vi "Модификация Витерби.vi"(7 "Кадр с мягкими\nзначениями":dbl[](array[numeric])) -> (8 "Декодированный поток битов":bool[](array[boolean]))   [LabVIEW 2013]
panel:
  in  "Array":cluster{bool, bool}[](array[cluster])=[{TRUE, TRUE}, {TRUE, FALSE}, {FALSE, TRUE}, {FALSE, FALSE}]
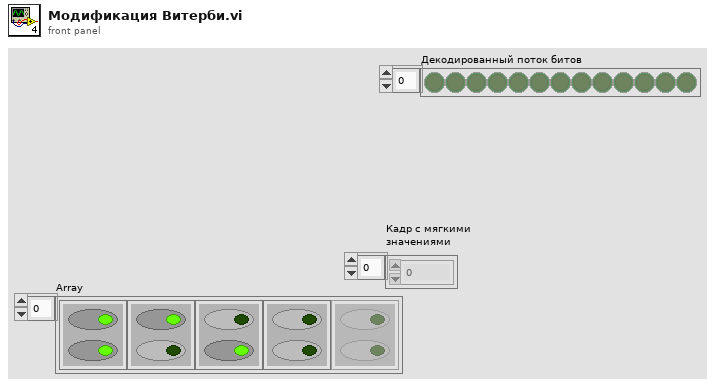
[diagram p1: front panel]
types:
  T1 = cluster{"Пр сост0":i32, "Ном зн\nреб0":i32, "Пр сост1":i32, "Ном зн\nреб1":i32, "Бит":bool}[]
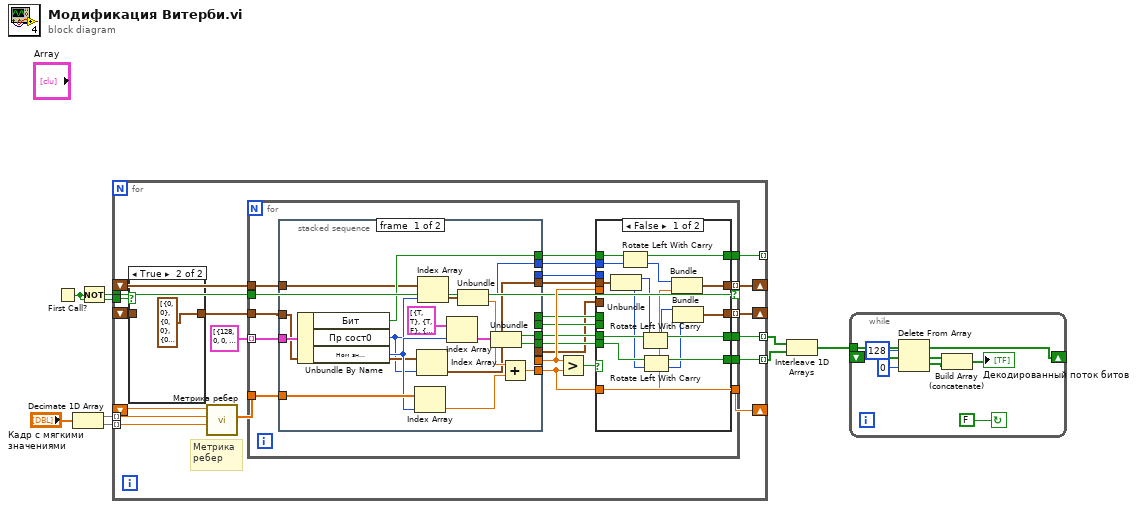
[diagram p0: block diagram]
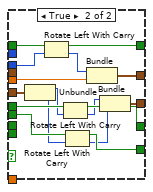
[diagram p3: hidden frame]
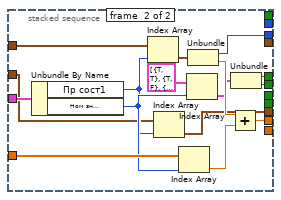
[diagram p4: hidden frame]
diagram:
  n1 = First Call?() -> (First Call?: T/F=w1:bool)
  n2 = Decimate 1D Array("Кадр с мягкими\nзначениями") -> (w7:dbl[], w6:dbl[])
  n3 = Not(x=w1) -> (.not. x?=w5:bool)
  n4 = for {
    tunnel: w7 -> [w18] mode=indexing
    tunnel: w6 -> [w17] mode=indexing
    tunnel: [w23] -> _ mode=indexing
    shift-right: [w22] -> _
    shift-left: _ -> [w21]
    shift-right: [w20] -> _
    shift-left: _ -> [w19]
    tunnel: w5 -> [w15]
    tunnel: [w14] -> w3 mode=indexing
    tunnel: [w13] -> w4 mode=indexing
    shift-right: [w12] -> _
    shift-left: _ -> [w9]
    tunnel: w1 -> [w11]
    # "Метрика\nребер"
    n5 = case shown="True" w11 {
      tunnel: [w25 cluster{u64, u64}[] [{0, 0}, {0, 0}, {0, 0}, {0, 0}, {0, 0}, {0, 0}, {0, 0}, {0, 0}, {0, 0}, {0, 0}, {0, 0}, {0, 0}, {0, 0}, {0, 0}, {0, 0}, {0, 0}, {0, 0}, {0, 0}, {0, 0}, {0, 0}, {0, 0}, {0, 0}, {0, 0}, {0, 0}, {0, 0}, {0, 0}, {0, 0}, {0, 0}, {0, 0}, {0, 0}, {0, 0}, {0, 0}, {0, 0}, {0, 0}, {0, 0}, {0, 0}, {0, 0}, {0, 0}, {0, 0}, {0, 0}, {0, 0}, {0, 0}, {0, 0}, {0, 0}, {0, 0}, {0, 0}, {0, 0}, {0, 0}, {0, 0}, {0, 0}, {0, 0}, {0, 0}, {0, 0}, {0, 0}, {0, 0}, {0, 0}, {0, 0}, {0, 0}, {0, 0}, {0, 0}, {0, 0}, {0, 0}, {0, 0}, {0, 0}, {0, 0}, {0, 0}, {0, 0}, {0, 0}, {0, 0}, {0, 0}, {0, 0}, {0, 0}, {0, 0}, {0, 0}, {0, 0}, {0, 0}, {0, 0}, {0, 0}, {0, 0}, {0, 0}, {0, 0}, {0, 0}, {0, 0}, {0, 0}, {0, 0}, {0, 0}, {0, 0}, {0, 0}, {0, 0}, {0, 0}, {0, 0}, {0, 0}, {0, 0}, {0, 0}, {0, 0}, {0, 0}, {0, 0}, {0, 0}, {0, 0}, {0, 0}, {0, 0}, {0, 0}, {0, 0}, {0, 0}, {0, 0}, {0, 0}, {0, 0}, {0, 0}, {0, 0}, {0, 0}, {0, 0}, {0, 0}, {0, 0}, {0, 0}, {0, 0}, {0, 0}, {0, 0}, {0, 0}, {0, 0}, {0, 0}, {0, 0}, {0, 0}, {0, 0}, {0, 0}, {0, 0}, {0, 0}, {0, 0}, {0, 0}, {0, 0}, {0, 0}, {0, 0}, {0, 0}, {0, 0}, {0, 0}, {0, 0}, {0, 0}, {0, 0}, {0, 0}, {0, 0}, {0, 0}, {0, 0}, {0, 0}, {0, 0}, {0, 0}, {0, 0}, {0, 0}, {0, 0}, {0, 0}, {0, 0}, {0, 0}, {0, 0}, {0, 0}, {0, 0}, {0, 0}, {0, 0}, {0, 0}, {0, 0}, {0, 0}, {0, 0}, {0, 0}, {0, 0}, {0, 0}, {0, 0}, {0, 0}, {0, 0}, {0, 0}, {0, 0}, {0, 0}, {0, 0}, {0, 0}, {0, 0}, {0, 0}, {0, 0}, {0, 0}, {0, 0}, {0, 0}, {0, 0}, {0, 0}, {0, 0}, {0, 0}, {0, 0}, {0, 0}, {0, 0}, {0, 0}, {0, 0}, {0, 0}, {0, 0}, {0, 0}, {0, 0}, {0, 0}, {0, 0}, {0, 0}, {0, 0}, {0, 0}, {0, 0}, {0, 0}, {0, 0}, {0, 0}, {0, 0}, {0, 0}, {0, 0}, {0, 0}, {0, 0}, {0, 0}, {0, 0}, {0, 0}, {0, 0}, {0, 0}, {0, 0}, {0, 0}, {0, 0}, {0, 0}, {0, 0}, {0, 0}, {0, 0}, {0, 0}, {0, 0}, {0, 0}, {0, 0}, {0, 0}, {0, 0}, {0, 0}, {0, 0}, {0, 0}, {0, 0}, {0, 0}, {0, 0}, {0, 0}, {0, 0}, {0, 0}, {0, 0}, {0, 0}, {0, 0}, {0, 0}, {0, 0}, {0, 0}, {0, 0}, {0, 0}, {0, 0}, {0, 0}, {0, 0}, {0, 0}, {0, 0}, {0, 0}, {0, 0}, {0, 0}, {0, 0}, {0, 0}, {0, 0}, {0, 0}, {0, 0}, {0, 0}, {0, 0}, {0, 0}, {0, 0}, {0, 0}]] -> w10
      tunnel: w9 -> [w25 _]
      frame False {
      }
      frame True {
      }
    }
    n6 = call "Метрика ребер.vi"("Бит неч"=w17, "Бит чет"=w18, "ПОРОГ"=w19) -> ("Возможные\nметрики ребер"=w24:dbl[])  [unwired: 8 in]
    n7 = for {
      tunnel: T1 [{"Пр сост0"=128, "Ном зн\nреб0"=0, "Пр сост1"=0, "Ном зн\nреб1"=3, "Бит"=FALSE}, {"Пр сост0"=128, "Ном зн\nреб0"=3, "Пр сост1"=0, "Ном зн\nреб1"=0, "Бит"=TRUE}, {"Пр сост0"=129, "Ном зн\nреб0"=1, "Пр сост1"=1, "Ном зн\nреб1"=2, "Бит"=FALSE}, {"Пр сост0"=129, "Ном зн\nреб0"=2, "Пр сост1"=1, "Ном зн\nреб1"=1, "Бит"=TRUE}, {"Пр сост0"=130, "Ном зн\nреб0"=3, "Пр сост1"=2, "Ном зн\nреб1"=0, "Бит"=FALSE}, {"Пр сост0"=130, "Ном зн\nреб0"=0, "Пр сост1"=2, "Ном зн\nреб1"=3, "Бит"=TRUE}, {"Пр сост0"=131, "Ном зн\nреб0"=2, "Пр сост1"=3, "Ном зн\nреб1"=1, "Бит"=FALSE}, {"Пр сост0"=131, "Ном зн\nреб0"=1, "Пр сост1"=3, "Ном зн\nреб1"=2, "Бит"=TRUE}, {"Пр сост0"=132, "Ном зн\nреб0"=3, "Пр сост1"=4, "Ном зн\nреб1"=0, "Бит"=FALSE}, {"Пр сост0"=132, "Ном зн\nреб0"=0, "Пр сост1"=4, "Ном зн\nреб1"=3, "Бит"=TRUE}, {"Пр сост0"=133, "Ном зн\nреб0"=2, "Пр сост1"=5, "Ном зн\nреб1"=1, "Бит"=FALSE}, {"Пр сост0"=133, "Ном зн\nреб0"=1, "Пр сост1"=5, "Ном зн\nреб1"=2, "Бит"=TRUE}, {"Пр сост0"=134, "Ном зн\nреб0"=0, "Пр сост1"=6, "Ном зн\nреб1"=3, "Бит"=FALSE}, {"Пр сост0"=134, "Ном зн\nреб0"=3, "Пр сост1"=6, "Ном зн\nреб1"=0, "Бит"=TRUE}, {"Пр сост0"=135, "Ном зн\nреб0"=1, "Пр сост1"=7, "Ном зн\nреб1"=2, "Бит"=FALSE}, {"Пр сост0"=135, "Ном зн\nреб0"=2, "Пр сост1"=7, "Ном зн\nреб1"=1, "Бит"=TRUE}, {"Пр сост0"=136, "Ном зн\nреб0"=2, "Пр сост1"=8, "Ном зн\nреб1"=1, "Бит"=FALSE}, {"Пр сост0"=136, "Ном зн\nреб0"=1, "Пр сост1"=8, "Ном зн\nреб1"=2, "Бит"=TRUE}, {"Пр сост0"=137, "Ном зн\nреб0"=3, "Пр сост1"=9, "Ном зн\nреб1"=0, "Бит"=FALSE}, {"Пр сост0"=137, "Ном зн\nреб0"=0, "Пр сост1"=9, "Ном зн\nреб1"=3, "Бит"=TRUE}, {"Пр сост0"=138, "Ном зн\nреб0"=1, "Пр сост1"=10, "Ном зн\nреб1"=2, "Бит"=FALSE}, {"Пр сост0"=138, "Ном зн\nреб0"=2, "Пр сост1"=10, "Ном зн\nреб1"=1, "Бит"=TRUE}, {"Пр сост0"=139, "Ном зн\nреб0"=0, "Пр сост1"=11, "Ном зн\nреб1"=3, "Бит"=FALSE}, {"Пр сост0"=139, "Ном зн\nреб0"=3, "Пр сост1"=11, "Ном зн\nреб1"=0, "Бит"=TRUE}, {"Пр сост0"=140, "Ном зн\nреб0"=1, "Пр сост1"=12, "Ном зн\nреб1"=2, "Бит"=FALSE}, {"Пр сост0"=140, "Ном зн\nреб0"=2, "Пр сост1"=12, "Ном зн\nреб1"=1, "Бит"=TRUE}, {"Пр сост0"=141, "Ном зн\nреб0"=0, "Пр сост1"=13, "Ном зн\nреб1"=3, "Бит"=FALSE}, {"Пр сост0"=141, "Ном зн\nреб0"=3, "Пр сост1"=13, "Ном зн\nреб1"=0, "Бит"=TRUE}, {"Пр сост0"=142, "Ном зн\nреб0"=2, "Пр сост1"=14, "Ном зн\nреб1"=1, "Бит"=FALSE}, {"Пр сост0"=142, "Ном зн\nреб0"=1, "Пр сост1"=14, "Ном зн\nреб1"=2, "Бит"=TRUE}, {"Пр сост0"=143, "Ном зн\nреб0"=3, "Пр сост1"=15, "Ном зн\nреб1"=0, "Бит"=FALSE}, {"Пр сост0"=143, "Ном зн\nреб0"=0, "Пр сост1"=15, "Ном зн\nреб1"=3, "Бит"=TRUE}, {"Пр сост0"=144, "Ном зн\nреб0"=1, "Пр сост1"=16, "Ном зн\nреб1"=2, "Бит"=FALSE}, {"Пр сост0"=144, "Ном зн\nреб0"=2, "Пр сост1"=16, "Ном зн\nреб1"=1, "Бит"=TRUE}, {"Пр сост0"=145, "Ном зн\nреб0"=0, "Пр сост1"=17, "Ном зн\nреб1"=3, "Бит"=FALSE}, {"Пр сост0"=145, "Ном зн\nреб0"=3, "Пр сост1"=17, "Ном зн\nреб1"=0, "Бит"=TRUE}, {"Пр сост0"=146, "Ном зн\nреб0"=2, "Пр сост1"=18, "Ном зн\nреб1"=1, "Бит"=FALSE}, {"Пр сост0"=146, "Ном зн\nреб0"=1, "Пр сост1"=18, "Ном зн\nреб1"=2, "Бит"=TRUE}, {"Пр сост0"=147, "Ном зн\nреб0"=3, "Пр сост1"=19, "Ном зн\nреб1"=0, "Бит"=FALSE}, {"Пр сост0"=147, "Ном зн\nреб0"=0, "Пр сост1"=19, "Ном зн\nреб1"=3, "Бит"=TRUE}, {"Пр сост0"=148, "Ном зн\nреб0"=2, "Пр сост1"=20, "Ном зн\nреб1"=1, "Бит"=FALSE}, {"Пр сост0"=148, "Ном зн\nреб0"=1, "Пр сост1"=20, "Ном зн\nреб1"=2, "Бит"=TRUE}, {"Пр сост0"=149, "Ном зн\nреб0"=3, "Пр сост1"=21, "Ном зн\nреб1"=0, "Бит"=FALSE}, {"Пр сост0"=149, "Ном зн\nреб0"=0, "Пр сост1"=21, "Ном зн\nреб1"=3, "Бит"=TRUE}, {"Пр сост0"=150, "Ном зн\nреб0"=1, "Пр сост1"=22, "Ном зн\nреб1"=2, "Бит"=FALSE}, {"Пр сост0"=150, "Ном зн\nреб0"=2, "Пр сост1"=22, "Ном зн\nреб1"=1, "Бит"=TRUE}, {"Пр сост0"=151, "Ном зн\nреб0"=0, "Пр сост1"=23, "Ном зн\nреб1"=3, "Бит"=FALSE}, {"Пр сост0"=151, "Ном зн\nреб0"=3, "Пр сост1"=23, "Ном зн\nреб1"=0, "Бит"=TRUE}, {"Пр сост0"=152, "Ном зн\nреб0"=3, "Пр сост1"=24, "Ном зн\nреб1"=0, "Бит"=FALSE}, {"Пр сост0"=152, "Ном зн\nреб0"=0, "Пр сост1"=24, "Ном зн\nреб1"=3, "Бит"=TRUE}, {"Пр сост0"=153, "Ном зн\nреб0"=2, "Пр сост1"=25, "Ном зн\nреб1"=1, "Бит"=FALSE}, {"Пр сост0"=153, "Ном зн\nреб0"=1, "Пр сост1"=25, "Ном зн\nреб1"=2, "Бит"=TRUE}, {"Пр сост0"=154, "Ном зн\nреб0"=0, "Пр сост1"=26, "Ном зн\nреб1"=3, "Бит"=FALSE}, {"Пр сост0"=154, "Ном зн\nреб0"=3, "Пр сост1"=26, "Ном зн\nреб1"=0, "Бит"=TRUE}, {"Пр сост0"=155, "Ном зн\nреб0"=1, "Пр сост1"=27, "Ном зн\nреб1"=2, "Бит"=FALSE}, {"Пр сост0"=155, "Ном зн\nреб0"=2, "Пр сост1"=27, "Ном зн\nреб1"=1, "Бит"=TRUE}, {"Пр сост0"=156, "Ном зн\nреб0"=0, "Пр сост1"=28, "Ном зн\nреб1"=3, "Бит"=FALSE}, {"Пр сост0"=156, "Ном зн\nреб0"=3, "Пр сост1"=28, "Ном зн\nреб1"=0, "Бит"=TRUE}, {"Пр сост0"=157, "Ном зн\nреб0"=1, "Пр сост1"=29, "Ном зн\nреб1"=2, "Бит"=FALSE}, {"Пр сост0"=157, "Ном зн\nреб0"=2, "Пр сост1"=29, "Ном зн\nреб1"=1, "Бит"=TRUE}, {"Пр сост0"=158, "Ном зн\nреб0"=3, "Пр сост1"=30, "Ном зн\nреб1"=0, "Бит"=FALSE}, {"Пр сост0"=158, "Ном зн\nреб0"=0, "Пр сост1"=30, "Ном зн\nреб1"=3, "Бит"=TRUE}, {"Пр сост0"=159, "Ном зн\nреб0"=2, "Пр сост1"=31, "Ном зн\nреб1"=1, "Бит"=FALSE}, {"Пр сост0"=159, "Ном зн\nреб0"=1, "Пр сост1"=31, "Ном зн\nреб1"=2, "Бит"=TRUE}, {"Пр сост0"=160, "Ном зн\nреб0"=0, "Пр сост1"=32, "Ном зн\nреб1"=3, "Бит"=FALSE}, {"Пр сост0"=160, "Ном зн\nреб0"=3, "Пр сост1"=32, "Ном зн\nреб1"=0, "Бит"=TRUE}, {"Пр сост0"=161, "Ном зн\nреб0"=1, "Пр сост1"=33, "Ном зн\nреб1"=2, "Бит"=FALSE}, {"Пр сост0"=161, "Ном зн\nреб0"=2, "Пр сост1"=33, "Ном зн\nреб1"=1, "Бит"=TRUE}, {"Пр сост0"=162, "Ном зн\nреб0"=3, "Пр сост1"=34, "Ном зн\nреб1"=0, "Бит"=FALSE}, {"Пр сост0"=162, "Ном зн\nреб0"=0, "Пр сост1"=34, "Ном зн\nреб1"=3, "Бит"=TRUE}, {"Пр сост0"=163, "Ном зн\nреб0"=2, "Пр сост1"=35, "Ном зн\nреб1"=1, "Бит"=FALSE}, {"Пр сост0"=163, "Ном зн\nреб0"=1, "Пр сост1"=35, "Ном зн\nреб1"=2, "Бит"=TRUE}, {"Пр сост0"=164, "Ном зн\nреб0"=3, "Пр сост1"=36, "Ном зн\nреб1"=0, "Бит"=FALSE}, {"Пр сост0"=164, "Ном зн\nреб0"=0, "Пр сост1"=36, "Ном зн\nреб1"=3, "Бит"=TRUE}, {"Пр сост0"=165, "Ном зн\nреб0"=2, "Пр сост1"=37, "Ном зн\nреб1"=1, "Бит"=FALSE}, {"Пр сост0"=165, "Ном зн\nреб0"=1, "Пр сост1"=37, "Ном зн\nреб1"=2, "Бит"=TRUE}, {"Пр сост0"=166, "Ном зн\nреб0"=0, "Пр сост1"=38, "Ном зн\nреб1"=3, "Бит"=FALSE}, {"Пр сост0"=166, "Ном зн\nреб0"=3, "Пр сост1"=38, "Ном зн\nреб1"=0, "Бит"=TRUE}, {"Пр сост0"=167, "Ном зн\nреб0"=1, "Пр сост1"=39, "Ном зн\nреб1"=2, "Бит"=FALSE}, {"Пр сост0"=167, "Ном зн\nреб0"=2, "Пр сост1"=39, "Ном зн\nреб1"=1, "Бит"=TRUE}, {"Пр сост0"=168, "Ном зн\nреб0"=2, "Пр сост1"=40, "Ном зн\nреб1"=1, "Бит"=FALSE}, {"Пр сост0"=168, "Ном зн\nреб0"=1, "Пр сост1"=40, "Ном зн\nреб1"=2, "Бит"=TRUE}, {"Пр сост0"=169, "Ном зн\nреб0"=3, "Пр сост1"=41, "Ном зн\nреб1"=0, "Бит"=FALSE}, {"Пр сост0"=169, "Ном зн\nреб0"=0, "Пр сост1"=41, "Ном зн\nреб1"=3, "Бит"=TRUE}, {"Пр сост0"=170, "Ном зн\nреб0"=1, "Пр сост1"=42, "Ном зн\nреб1"=2, "Бит"=FALSE}, {"Пр сост0"=170, "Ном зн\nреб0"=2, "Пр сост1"=42, "Ном зн\nреб1"=1, "Бит"=TRUE}, {"Пр сост0"=171, "Ном зн\nреб0"=0, "Пр сост1"=43, "Ном зн\nреб1"=3, "Бит"=FALSE}, {"Пр сост0"=171, "Ном зн\nреб0"=3, "Пр сост1"=43, "Ном зн\nреб1"=0, "Бит"=TRUE}, {"Пр сост0"=172, "Ном зн\nреб0"=1, "Пр сост1"=44, "Ном зн\nреб1"=2, "Бит"=FALSE}, {"Пр сост0"=172, "Ном зн\nреб0"=2, "Пр сост1"=44, "Ном зн\nреб1"=1, "Бит"=TRUE}, {"Пр сост0"=173, "Ном зн\nреб0"=0, "Пр сост1"=45, "Ном зн\nреб1"=3, "Бит"=FALSE}, {"Пр сост0"=173, "Ном зн\nреб0"=3, "Пр сост1"=45, "Ном зн\nреб1"=0, "Бит"=TRUE}, {"Пр сост0"=174, "Ном зн\nреб0"=2, "Пр сост1"=46, "Ном зн\nреб1"=1, "Бит"=FALSE}, {"Пр сост0"=174, "Ном зн\nреб0"=1, "Пр сост1"=46, "Ном зн\nреб1"=2, "Бит"=TRUE}, {"Пр сост0"=175, "Ном зн\nреб0"=3, "Пр сост1"=47, "Ном зн\nреб1"=0, "Бит"=FALSE}, {"Пр сост0"=175, "Ном зн\nреб0"=0, "Пр сост1"=47, "Ном зн\nреб1"=3, "Бит"=TRUE}, {"Пр сост0"=176, "Ном зн\nреб0"=1, "Пр сост1"=48, "Ном зн\nреб1"=2, "Бит"=FALSE}, {"Пр сост0"=176, "Ном зн\nреб0"=2, "Пр сост1"=48, "Ном зн\nреб1"=1, "Бит"=TRUE}, {"Пр сост0"=177, "Ном зн\nреб0"=0, "Пр сост1"=49, "Ном зн\nреб1"=3, "Бит"=FALSE}, {"Пр сост0"=177, "Ном зн\nреб0"=3, "Пр сост1"=49, "Ном зн\nреб1"=0, "Бит"=TRUE}, {"Пр сост0"=178, "Ном зн\nреб0"=2, "Пр сост1"=50, "Ном зн\nреб1"=1, "Бит"=FALSE}, {"Пр сост0"=178, "Ном зн\nреб0"=1, "Пр сост1"=50, "Ном зн\nреб1"=2, "Бит"=TRUE}, {"Пр сост0"=179, "Ном зн\nреб0"=3, "Пр сост1"=51, "Ном зн\nреб1"=0, "Бит"=FALSE}, {"Пр сост0"=179, "Ном зн\nреб0"=0, "Пр сост1"=51, "Ном зн\nреб1"=3, "Бит"=TRUE}, {"Пр сост0"=180, "Ном зн\nреб0"=2, "Пр сост1"=52, "Ном зн\nреб1"=1, "Бит"=FALSE}, {"Пр сост0"=180, "Ном зн\nреб0"=1, "Пр сост1"=52, "Ном зн\nреб1"=2, "Бит"=TRUE}, {"Пр сост0"=181, "Ном зн\nреб0"=3, "Пр сост1"=53, "Ном зн\nреб1"=0, "Бит"=FALSE}, {"Пр сост0"=181, "Ном зн\nреб0"=0, "Пр сост1"=53, "Ном зн\nреб1"=3, "Бит"=TRUE}, {"Пр сост0"=182, "Ном зн\nреб0"=1, "Пр сост1"=54, "Ном зн\nреб1"=2, "Бит"=FALSE}, {"Пр сост0"=182, "Ном зн\nреб0"=2, "Пр сост1"=54, "Ном зн\nреб1"=1, "Бит"=TRUE}, {"Пр сост0"=183, "Ном зн\nреб0"=0, "Пр сост1"=55, "Ном зн\nреб1"=3, "Бит"=FALSE}, {"Пр сост0"=183, "Ном зн\nреб0"=3, "Пр сост1"=55, "Ном зн\nреб1"=0, "Бит"=TRUE}, {"Пр сост0"=184, "Ном зн\nреб0"=3, "Пр сост1"=56, "Ном зн\nреб1"=0, "Бит"=FALSE}, {"Пр сост0"=184, "Ном зн\nреб0"=0, "Пр сост1"=56, "Ном зн\nреб1"=3, "Бит"=TRUE}, {"Пр сост0"=185, "Ном зн\nреб0"=2, "Пр сост1"=57, "Ном зн\nреб1"=1, "Бит"=FALSE}, {"Пр сост0"=185, "Ном зн\nреб0"=1, "Пр сост1"=57, "Ном зн\nреб1"=2, "Бит"=TRUE}, {"Пр сост0"=186, "Ном зн\nреб0"=0, "Пр сост1"=58, "Ном зн\nреб1"=3, "Бит"=FALSE}, {"Пр сост0"=186, "Ном зн\nреб0"=3, "Пр сост1"=58, "Ном зн\nреб1"=0, "Бит"=TRUE}, {"Пр сост0"=187, "Ном зн\nреб0"=1, "Пр сост1"=59, "Ном зн\nреб1"=2, "Бит"=FALSE}, {"Пр сост0"=187, "Ном зн\nреб0"=2, "Пр сост1"=59, "Ном зн\nреб1"=1, "Бит"=TRUE}, {"Пр сост0"=188, "Ном зн\nреб0"=0, "Пр сост1"=60, "Ном зн\nреб1"=3, "Бит"=FALSE}, {"Пр сост0"=188, "Ном зн\nреб0"=3, "Пр сост1"=60, "Ном зн\nреб1"=0, "Бит"=TRUE}, {"Пр сост0"=189, "Ном зн\nреб0"=1, "Пр сост1"=61, "Ном зн\nреб1"=2, "Бит"=FALSE}, {"Пр сост0"=189, "Ном зн\nреб0"=2, "Пр сост1"=61, "Ном зн\nреб1"=1, "Бит"=TRUE}, {"Пр сост0"=190, "Ном зн\nреб0"=3, "Пр сост1"=62, "Ном зн\nреб1"=0, "Бит"=FALSE}, {"Пр сост0"=190, "Ном зн\nреб0"=0, "Пр сост1"=62, "Ном зн\nреб1"=3, "Бит"=TRUE}, {"Пр сост0"=191, "Ном зн\nреб0"=2, "Пр сост1"=63, "Ном зн\nреб1"=1, "Бит"=FALSE}, {"Пр сост0"=191, "Ном зн\nреб0"=1, "Пр сост1"=63, "Ном зн\nреб1"=2, "Бит"=TRUE}, {"Пр сост0"=192, "Ном зн\nреб0"=1, "Пр сост1"=64, "Ном зн\nреб1"=2, "Бит"=FALSE}, {"Пр сост0"=192, "Ном зн\nреб0"=2, "Пр сост1"=64, "Ном зн\nреб1"=1, "Бит"=TRUE}, {"Пр сост0"=193, "Ном зн\nреб0"=0, "Пр сост1"=65, "Ном зн\nреб1"=3, "Бит"=FALSE}, {"Пр сост0"=193, "Ном зн\nреб0"=3, "Пр сост1"=65, "Ном зн\nреб1"=0, "Бит"=TRUE}, {"Пр сост0"=194, "Ном зн\nреб0"=2, "Пр сост1"=66, "Ном зн\nреб1"=1, "Бит"=FALSE}, {"Пр сост0"=194, "Ном зн\nреб0"=1, "Пр сост1"=66, "Ном зн\nреб1"=2, "Бит"=TRUE}, {"Пр сост0"=195, "Ном зн\nреб0"=3, "Пр сост1"=67, "Ном зн\nреб1"=0, "Бит"=FALSE}, {"Пр сост0"=195, "Ном зн\nреб0"=0, "Пр сост1"=67, "Ном зн\nреб1"=3, "Бит"=TRUE}, {"Пр сост0"=196, "Ном зн\nреб0"=2, "Пр сост1"=68, "Ном зн\nреб1"=1, "Бит"=FALSE}, {"Пр сост0"=196, "Ном зн\nреб0"=1, "Пр сост1"=68, "Ном зн\nреб1"=2, "Бит"=TRUE}, {"Пр сост0"=197, "Ном зн\nреб0"=3, "Пр сост1"=69, "Ном зн\nреб1"=0, "Бит"=FALSE}, {"Пр сост0"=197, "Ном зн\nреб0"=0, "Пр сост1"=69, "Ном зн\nреб1"=3, "Бит"=TRUE}, {"Пр сост0"=198, "Ном зн\nреб0"=1, "Пр сост1"=70, "Ном зн\nреб1"=2, "Бит"=FALSE}, {"Пр сост0"=198, "Ном зн\nреб0"=2, "Пр сост1"=70, "Ном зн\nреб1"=1, "Бит"=TRUE}, {"Пр сост0"=199, "Ном зн\nреб0"=0, "Пр сост1"=71, "Ном зн\nреб1"=3, "Бит"=FALSE}, {"Пр сост0"=199, "Ном зн\nреб0"=3, "Пр сост1"=71, "Ном зн\nреб1"=0, "Бит"=TRUE}, {"Пр сост0"=200, "Ном зн\nреб0"=3, "Пр сост1"=72, "Ном зн\nреб1"=0, "Бит"=FALSE}, {"Пр сост0"=200, "Ном зн\nреб0"=0, "Пр сост1"=72, "Ном зн\nреб1"=3, "Бит"=TRUE}, {"Пр сост0"=201, "Ном зн\nреб0"=2, "Пр сост1"=73, "Ном зн\nреб1"=1, "Бит"=FALSE}, {"Пр сост0"=201, "Ном зн\nреб0"=1, "Пр сост1"=73, "Ном зн\nреб1"=2, "Бит"=TRUE}, {"Пр сост0"=202, "Ном зн\nреб0"=0, "Пр сост1"=74, "Ном зн\nреб1"=3, "Бит"=FALSE}, {"Пр сост0"=202, "Ном зн\nреб0"=3, "Пр сост1"=74, "Ном зн\nреб1"=0, "Бит"=TRUE}, {"Пр сост0"=203, "Ном зн\nреб0"=1, "Пр сост1"=75, "Ном зн\nреб1"=2, "Бит"=FALSE}, {"Пр сост0"=203, "Ном зн\nреб0"=2, "Пр сост1"=75, "Ном зн\nреб1"=1, "Бит"=TRUE}, {"Пр сост0"=204, "Ном зн\nреб0"=0, "Пр сост1"=76, "Ном зн\nреб1"=3, "Бит"=FALSE}, {"Пр сост0"=204, "Ном зн\nреб0"=3, "Пр сост1"=76, "Ном зн\nреб1"=0, "Бит"=TRUE}, {"Пр сост0"=205, "Ном зн\nреб0"=1, "Пр сост1"=77, "Ном зн\nреб1"=2, "Бит"=FALSE}, {"Пр сост0"=205, "Ном зн\nреб0"=2, "Пр сост1"=77, "Ном зн\nреб1"=1, "Бит"=TRUE}, {"Пр сост0"=206, "Ном зн\nреб0"=3, "Пр сост1"=78, "Ном зн\nреб1"=0, "Бит"=FALSE}, {"Пр сост0"=206, "Ном зн\nреб0"=0, "Пр сост1"=78, "Ном зн\nреб1"=3, "Бит"=TRUE}, {"Пр сост0"=207, "Ном зн\nреб0"=2, "Пр сост1"=79, "Ном зн\nреб1"=1, "Бит"=FALSE}, {"Пр сост0"=207, "Ном зн\nреб0"=1, "Пр сост1"=79, "Ном зн\nреб1"=2, "Бит"=TRUE}, {"Пр сост0"=208, "Ном зн\nреб0"=0, "Пр сост1"=80, "Ном зн\nреб1"=3, "Бит"=FALSE}, {"Пр сост0"=208, "Ном зн\nреб0"=3, "Пр сост1"=80, "Ном зн\nреб1"=0, "Бит"=TRUE}, {"Пр сост0"=209, "Ном зн\nреб0"=1, "Пр сост1"=81, "Ном зн\nреб1"=2, "Бит"=FALSE}, {"Пр сост0"=209, "Ном зн\nреб0"=2, "Пр сост1"=81, "Ном зн\nреб1"=1, "Бит"=TRUE}, {"Пр сост0"=210, "Ном зн\nреб0"=3, "Пр сост1"=82, "Ном зн\nреб1"=0, "Бит"=FALSE}, {"Пр сост0"=210, "Ном зн\nреб0"=0, "Пр сост1"=82, "Ном зн\nреб1"=3, "Бит"=TRUE}, {"Пр сост0"=211, "Ном зн\nреб0"=2, "Пр сост1"=83, "Ном зн\nреб1"=1, "Бит"=FALSE}, {"Пр сост0"=211, "Ном зн\nреб0"=1, "Пр сост1"=83, "Ном зн\nреб1"=2, "Бит"=TRUE}, {"Пр сост0"=212, "Ном зн\nреб0"=3, "Пр сост1"=84, "Ном зн\nреб1"=0, "Бит"=FALSE}, {"Пр сост0"=212, "Ном зн\nреб0"=0, "Пр сост1"=84, "Ном зн\nреб1"=3, "Бит"=TRUE}, {"Пр сост0"=213, "Ном зн\nреб0"=2, "Пр сост1"=85, "Ном зн\nреб1"=1, "Бит"=FALSE}, {"Пр сост0"=213, "Ном зн\nреб0"=1, "Пр сост1"=85, "Ном зн\nреб1"=2, "Бит"=TRUE}, {"Пр сост0"=214, "Ном зн\nреб0"=0, "Пр сост1"=86, "Ном зн\nреб1"=3, "Бит"=FALSE}, {"Пр сост0"=214, "Ном зн\nреб0"=3, "Пр сост1"=86, "Ном зн\nреб1"=0, "Бит"=TRUE}, {"Пр сост0"=215, "Ном зн\nреб0"=1, "Пр сост1"=87, "Ном зн\nреб1"=2, "Бит"=FALSE}, {"Пр сост0"=215, "Ном зн\nреб0"=2, "Пр сост1"=87, "Ном зн\nреб1"=1, "Бит"=TRUE}, {"Пр сост0"=216, "Ном зн\nреб0"=2, "Пр сост1"=88, "Ном зн\nреб1"=1, "Бит"=FALSE}, {"Пр сост0"=216, "Ном зн\nреб0"=1, "Пр сост1"=88, "Ном зн\nреб1"=2, "Бит"=TRUE}, {"Пр сост0"=217, "Ном зн\nреб0"=3, "Пр сост1"=89, "Ном зн\nреб1"=0, "Бит"=FALSE}, {"Пр сост0"=217, "Ном зн\nреб0"=0, "Пр сост1"=89, "Ном зн\nреб1"=3, "Бит"=TRUE}, {"Пр сост0"=218, "Ном зн\nреб0"=1, "Пр сост1"=90, "Ном зн\nреб1"=2, "Бит"=FALSE}, {"Пр сост0"=218, "Ном зн\nреб0"=2, "Пр сост1"=90, "Ном зн\nреб1"=1, "Бит"=TRUE}, {"Пр сост0"=219, "Ном зн\nреб0"=0, "Пр сост1"=91, "Ном зн\nреб1"=3, "Бит"=FALSE}, {"Пр сост0"=219, "Ном зн\nреб0"=3, "Пр сост1"=91, "Ном зн\nреб1"=0, "Бит"=TRUE}, {"Пр сост0"=220, "Ном зн\nреб0"=1, "Пр сост1"=92, "Ном зн\nреб1"=2, "Бит"=FALSE}, {"Пр сост0"=220, "Ном зн\nреб0"=2, "Пр сост1"=92, "Ном зн\nреб1"=1, "Бит"=TRUE}, {"Пр сост0"=221, "Ном зн\nреб0"=0, "Пр сост1"=93, "Ном зн\nреб1"=3, "Бит"=FALSE}, {"Пр сост0"=221, "Ном зн\nреб0"=3, "Пр сост1"=93, "Ном зн\nреб1"=0, "Бит"=TRUE}, {"Пр сост0"=222, "Ном зн\nреб0"=2, "Пр сост1"=94, "Ном зн\nреб1"=1, "Бит"=FALSE}, {"Пр сост0"=222, "Ном зн\nреб0"=1, "Пр сост1"=94, "Ном зн\nреб1"=2, "Бит"=TRUE}, {"Пр сост0"=223, "Ном зн\nреб0"=3, "Пр сост1"=95, "Ном зн\nреб1"=0, "Бит"=FALSE}, {"Пр сост0"=223, "Ном зн\nреб0"=0, "Пр сост1"=95, "Ном зн\nреб1"=3, "Бит"=TRUE}, {"Пр сост0"=224, "Ном зн\nреб0"=1, "Пр сост1"=96, "Ном зн\nреб1"=2, "Бит"=FALSE}, {"Пр сост0"=224, "Ном зн\nреб0"=2, "Пр сост1"=96, "Ном зн\nреб1"=1, "Бит"=TRUE}, {"Пр сост0"=225, "Ном зн\nреб0"=0, "Пр сост1"=97, "Ном зн\nреб1"=3, "Бит"=FALSE}, {"Пр сост0"=225, "Ном зн\nреб0"=3, "Пр сост1"=97, "Ном зн\nреб1"=0, "Бит"=TRUE}, {"Пр сост0"=226, "Ном зн\nреб0"=2, "Пр сост1"=98, "Ном зн\nреб1"=1, "Бит"=FALSE}, {"Пр сост0"=226, "Ном зн\nреб0"=1, "Пр сост1"=98, "Ном зн\nреб1"=2, "Бит"=TRUE}, {"Пр сост0"=227, "Ном зн\nреб0"=3, "Пр сост1"=99, "Ном зн\nреб1"=0, "Бит"=FALSE}, {"Пр сост0"=227, "Ном зн\nреб0"=0, "Пр сост1"=99, "Ном зн\nреб1"=3, "Бит"=TRUE}, {"Пр сост0"=228, "Ном зн\nреб0"=2, "Пр сост1"=100, "Ном зн\nреб1"=1, "Бит"=FALSE}, {"Пр сост0"=228, "Ном зн\nреб0"=1, "Пр сост1"=100, "Ном зн\nреб1"=2, "Бит"=TRUE}, {"Пр сост0"=229, "Ном зн\nреб0"=3, "Пр сост1"=101, "Ном зн\nреб1"=0, "Бит"=FALSE}, {"Пр сост0"=229, "Ном зн\nреб0"=0, "Пр сост1"=101, "Ном зн\nреб1"=3, "Бит"=TRUE}, {"Пр сост0"=230, "Ном зн\nреб0"=1, "Пр сост1"=102, "Ном зн\nреб1"=2, "Бит"=FALSE}, {"Пр сост0"=230, "Ном зн\nреб0"=2, "Пр сост1"=102, "Ном зн\nреб1"=1, "Бит"=TRUE}, {"Пр сост0"=231, "Ном зн\nреб0"=0, "Пр сост1"=103, "Ном зн\nреб1"=3, "Бит"=FALSE}, {"Пр сост0"=231, "Ном зн\nреб0"=3, "Пр сост1"=103, "Ном зн\nреб1"=0, "Бит"=TRUE}, {"Пр сост0"=232, "Ном зн\nреб0"=3, "Пр сост1"=104, "Ном зн\nреб1"=0, "Бит"=FALSE}, {"Пр сост0"=232, "Ном зн\nреб0"=0, "Пр сост1"=104, "Ном зн\nреб1"=3, "Бит"=TRUE}, {"Пр сост0"=233, "Ном зн\nреб0"=2, "Пр сост1"=105, "Ном зн\nреб1"=1, "Бит"=FALSE}, {"Пр сост0"=233, "Ном зн\nреб0"=1, "Пр сост1"=105, "Ном зн\nреб1"=2, "Бит"=TRUE}, {"Пр сост0"=234, "Ном зн\nреб0"=0, "Пр сост1"=106, "Ном зн\nреб1"=3, "Бит"=FALSE}, {"Пр сост0"=234, "Ном зн\nреб0"=3, "Пр сост1"=106, "Ном зн\nреб1"=0, "Бит"=TRUE}, {"Пр сост0"=235, "Ном зн\nреб0"=1, "Пр сост1"=107, "Ном зн\nреб1"=2, "Бит"=FALSE}, {"Пр сост0"=235, "Ном зн\nреб0"=2, "Пр сост1"=107, "Ном зн\nреб1"=1, "Бит"=TRUE}, {"Пр сост0"=236, "Ном зн\nреб0"=0, "Пр сост1"=108, "Ном зн\nреб1"=3, "Бит"=FALSE}, {"Пр сост0"=236, "Ном зн\nреб0"=3, "Пр сост1"=108, "Ном зн\nреб1"=0, "Бит"=TRUE}, {"Пр сост0"=237, "Ном зн\nреб0"=1, "Пр сост1"=109, "Ном зн\nреб1"=2, "Бит"=FALSE}, {"Пр сост0"=237, "Ном зн\nреб0"=2, "Пр сост1"=109, "Ном зн\nреб1"=1, "Бит"=TRUE}, {"Пр сост0"=238, "Ном зн\nреб0"=3, "Пр сост1"=110, "Ном зн\nреб1"=0, "Бит"=FALSE}, {"Пр сост0"=238, "Ном зн\nреб0"=0, "Пр сост1"=110, "Ном зн\nреб1"=3, "Бит"=TRUE}, {"Пр сост0"=239, "Ном зн\nреб0"=2, "Пр сост1"=111, "Ном зн\nреб1"=1, "Бит"=FALSE}, {"Пр сост0"=239, "Ном зн\nреб0"=1, "Пр сост1"=111, "Ном зн\nреб1"=2, "Бит"=TRUE}, {"Пр сост0"=240, "Ном зн\nреб0"=0, "Пр сост1"=112, "Ном зн\nреб1"=3, "Бит"=FALSE}, {"Пр сост0"=240, "Ном зн\nреб0"=3, "Пр сост1"=112, "Ном зн\nреб1"=0, "Бит"=TRUE}, {"Пр сост0"=241, "Ном зн\nреб0"=1, "Пр сост1"=113, "Ном зн\nреб1"=2, "Бит"=FALSE}, {"Пр сост0"=241, "Ном зн\nреб0"=2, "Пр сост1"=113, "Ном зн\nреб1"=1, "Бит"=TRUE}, {"Пр сост0"=242, "Ном зн\nреб0"=3, "Пр сост1"=114, "Ном зн\nреб1"=0, "Бит"=FALSE}, {"Пр сост0"=242, "Ном зн\nреб0"=0, "Пр сост1"=114, "Ном зн\nреб1"=3, "Бит"=TRUE}, {"Пр сост0"=243, "Ном зн\nреб0"=2, "Пр сост1"=115, "Ном зн\nреб1"=1, "Бит"=FALSE}, {"Пр сост0"=243, "Ном зн\nреб0"=1, "Пр сост1"=115, "Ном зн\nреб1"=2, "Бит"=TRUE}, {"Пр сост0"=244, "Ном зн\nреб0"=3, "Пр сост1"=116, "Ном зн\nреб1"=0, "Бит"=FALSE}, {"Пр сост0"=244, "Ном зн\nреб0"=0, "Пр сост1"=116, "Ном зн\nреб1"=3, "Бит"=TRUE}, {"Пр сост0"=245, "Ном зн\nреб0"=2, "Пр сост1"=117, "Ном зн\nреб1"=1, "Бит"=FALSE}, {"Пр сост0"=245, "Ном зн\nреб0"=1, "Пр сост1"=117, "Ном зн\nреб1"=2, "Бит"=TRUE}, {"Пр сост0"=246, "Ном зн\nреб0"=0, "Пр сост1"=118, "Ном зн\nреб1"=3, "Бит"=FALSE}, {"Пр сост0"=246, "Ном зн\nреб0"=3, "Пр сост1"=118, "Ном зн\nреб1"=0, "Бит"=TRUE}, {"Пр сост0"=247, "Ном зн\nреб0"=1, "Пр сост1"=119, "Ном зн\nреб1"=2, "Бит"=FALSE}, {"Пр сост0"=247, "Ном зн\nреб0"=2, "Пр сост1"=119, "Ном зн\nреб1"=1, "Бит"=TRUE}, {"Пр сост0"=248, "Ном зн\nреб0"=2, "Пр сост1"=120, "Ном зн\nреб1"=1, "Бит"=FALSE}, {"Пр сост0"=248, "Ном зн\nреб0"=1, "Пр сост1"=120, "Ном зн\nреб1"=2, "Бит"=TRUE}, {"Пр сост0"=249, "Ном зн\nреб0"=3, "Пр сост1"=121, "Ном зн\nреб1"=0, "Бит"=FALSE}, {"Пр сост0"=249, "Ном зн\nреб0"=0, "Пр сост1"=121, "Ном зн\nреб1"=3, "Бит"=TRUE}, {"Пр сост0"=250, "Ном зн\nреб0"=1, "Пр сост1"=122, "Ном зн\nреб1"=2, "Бит"=FALSE}, {"Пр сост0"=250, "Ном зн\nреб0"=2, "Пр сост1"=122, "Ном зн\nреб1"=1, "Бит"=TRUE}, {"Пр сост0"=251, "Ном зн\nреб0"=0, "Пр сост1"=123, "Ном зн\nреб1"=3, "Бит"=FALSE}, {"Пр сост0"=251, "Ном зн\nреб0"=3, "Пр сост1"=123, "Ном зн\nреб1"=0, "Бит"=TRUE}, {"Пр сост0"=252, "Ном зн\nреб0"=1, "Пр сост1"=124, "Ном зн\nреб1"=2, "Бит"=FALSE}, {"Пр сост0"=252, "Ном зн\nреб0"=2, "Пр сост1"=124, "Ном зн\nреб1"=1, "Бит"=TRUE}, {"Пр сост0"=253, "Ном зн\nреб0"=0, "Пр сост1"=125, "Ном зн\nреб1"=3, "Бит"=FALSE}, {"Пр сост0"=253, "Ном зн\nреб0"=3, "Пр сост1"=125, "Ном зн\nреб1"=0, "Бит"=TRUE}, {"Пр сост0"=254, "Ном зн\nреб0"=2, "Пр сост1"=126, "Ном зн\nреб1"=1, "Бит"=FALSE}, {"Пр сост0"=254, "Ном зн\nреб0"=1, "Пр сост1"=126, "Ном зн\nреб1"=2, "Бит"=TRUE}, {"Пр сост0"=255, "Ном зн\nреб0"=3, "Пр сост1"=127, "Ном зн\nреб1"=0, "Бит"=FALSE}, {"Пр сост0"=255, "Ном зн\nреб0"=0, "Пр сост1"=127, "Ном зн\nреб1"=3, "Бит"=TRUE}] ("Параметры метрики 2") -> [w48] mode=indexing
      tunnel: w24 -> [w47]
      tunnel: [w44] -> w23
      tunnel: [w42] -> w22 mode=indexing if=w37
      tunnel: w21 -> [w41]
      tunnel: [w38] -> w20
      tunnel: w15 -> [w37]
      tunnel: [w32] -> w14
      tunnel: [w31] -> w13
      tunnel: [w30] -> w12 mode=indexing
      tunnel: w10 -> [w29]
      n8 = stacked-sequence {
        tunnel: w48 -> [w97 w111]
        tunnel: w47 -> [w96 w112]
        tunnel: [w94 _] -> w38
        tunnel: [_ w110] -> w43
        tunnel: [w93 _] -> w45
        tunnel: w41 -> [w92 w108]
        tunnel: [w89 _] -> w40
        tunnel: [_ w106] -> w39
        tunnel: [w86 _] -> w36
        tunnel: [w85 _] -> w35
        tunnel: [_ w103] -> w34
        tunnel: [_ w102] -> w33
        tunnel: w29 -> [w83 w99]
        tunnel: [_ w98] -> w28
        tunnel: [w81 _] -> w27
        frame #0 {
          n9 = Unbundle By Name(w97) -> ("Бит"=w93:bool, "Пр сост0"=w82:i32, "Ном зн\nреб0"=w84:i32)
          n10 = Index Array(array=w96, index=w84) -> (element=w95:dbl)
          n11 = Index Array(array=w83, index=w82) -> (element=w81:cluster{u64, u64})
          n12 = Index Array(array=w92, index=w82) -> (element=w91:cluster{u64, dbl})
          n13 = Index Array(array=cluster{bool, bool}[] [{TRUE, TRUE}, {TRUE, FALSE}, {FALSE, TRUE}, {FALSE, FALSE}], index=w84) -> (element=w87:cluster{bool, bool})
          n14 = Unbundle(w91) -> (w89:u64, w90:dbl)
          n15 = Unbundle(w87) -> (w86:bool, w85:bool)
          n16 = Add(x=w90, y=w95) -> (x+y=w94:dbl)
        }
        frame #1 {
          n17 = Unbundle By Name(w111) -> ("Пр сост1"=w100:i32, "Ном зн\nреб1"=w101:i32)
          n18 = Index Array(array=w108, index=w100) -> (element=w109:cluster{u64, dbl})
          n19 = Index Array(array=w99, index=w100) -> (element=w98:cluster{u64, u64})
          n20 = Index Array(array=w112, index=w101) -> (element=w113:dbl)
          n21 = Index Array(array=cluster{bool, bool}[] [{TRUE, TRUE}, {TRUE, FALSE}, {FALSE, TRUE}, {FALSE, FALSE}], index=w101) -> (element=w105:cluster{bool, bool})
          n22 = Unbundle(w109) -> (w106:u64, w107:dbl)
          n23 = Add(x=w107, y=w113) -> (x+y=w110:dbl)
          n24 = Unbundle(w105) -> (w103:bool, w102:bool)
        }
      }
      n25 = Greater?(x=w43, y=w38) -> (0:w46:bool)
      n26 = case shown="False" w46 {
        tunnel: w45 -> [w63 w80]
        tunnel: [w62 w79] -> w44
        tunnel: w43 -> [_ w77]
        tunnel: [w61 w76] -> w42
        tunnel: w38 -> [w59 _]
        tunnel: w40 -> [w60 _]
        tunnel: w39 -> [_ w75]
        tunnel: w36 -> [w58 _]
        tunnel: w35 -> [w57 _]
        tunnel: w34 -> [_ w74]
        tunnel: w33 -> [_ w73]
        tunnel: [w56 w72] -> w31
        tunnel: [w55 w71] -> w32
        tunnel: [w54 w68] -> w30
        tunnel: w28 -> [_ w67]
        tunnel: w27 -> [w49 _]
        frame False {
          n27 = Unbundle(w49) -> (w51:u64, w50:u64)
          n28 = Rotate Left With Carry(2:w60, 3:w63) -> (0:w64:u64, 1:w62:bool)
          n29 = Rotate Left With Carry(2:w51, 3:w58) -> (0:w53:u64, 1:w56:bool)
          n30 = Rotate Left With Carry(2:w50, 3:w57) -> (0:w52:u64, 1:w55:bool)
          n31 = Bundle(w64, w59) -> (w61:cluster{u64, dbl})  [unwired: 1 in]
          n32 = Bundle(w53, w52) -> (w54:cluster{u64, u64})  [unwired: 1 in]
        }
        frame True {
          n33 = Unbundle(w67) -> (w66:u64, w65:u64)
          n34 = Rotate Left With Carry(2:w75, 3:w80) -> (0:w78:u64, 1:w79:bool)
          n35 = Rotate Left With Carry(2:w66, 3:w74) -> (0:w70:u64, 1:w72:bool)
          n36 = Rotate Left With Carry(2:w65, 3:w73) -> (0:w69:u64, 1:w71:bool)
          n37 = Bundle(w78, w77) -> (w76:cluster{u64, dbl})  [unwired: 1 in]
          n38 = Bundle(w70, w69) -> (w68:cluster{u64, u64})  [unwired: 1 in]
        }
      }
    }
  }
  n39 = Interleave 1D Arrays(w4, w3) -> (w2:bool[])
  n40 = while {
    tunnel: w2 -> [w121]
    shift-right: [w117] -> _
    shift-left: _ -> [w116]
    stop <- FALSE continue-if-true
    n41 = Delete From Array(array=w121, length=128, index=0) -> (deleted portion=w115:bool[], array with subset deleted=w117:bool[])
    n42 = Build Array (concatenate)(w116, w115) -> (→"Декодированный поток битов":bool[])
  }
